vi "LVClasse_SurfaceFloat GetStatisticDatas.vi"(0 "SurfaceFloat in":refnum<class "SurfaceFloat.lvclass">, 11 "error in (no error)":errorcluster) -> (4 "SurfaceFloat out":refnum<class "SurfaceFloat.lvclass">, 6 "StatisticsData":T1, 15 "error out":errorcluster)   [LabVIEW 2020, in "SurfaceFloat.lvclass"]
doc: "Get Surface statistics.\n\n--------------------------------------------------------------------------------\n\n<B>SurfaceIn </B> : Surface object.\n<B>SurfaceOut </B> : Surface object.\n<B>rms </B> : Surface root mean square deviation.\n<B>pv </B> : Surface peak to valley.\n<B>max </B> : Surface maximum.\n<B>min </B> : Surface minimum.\n<B>ErrorIn </B> : Error\n<B>ErrorOut </B> : Error\n\n--------------------------------------------------------------------------------"
uses:
  SurfaceFloat.lvclass
  StatisticsData.ctl
  SurfaceFloat.lvclass/SurfaceFloat.ctl
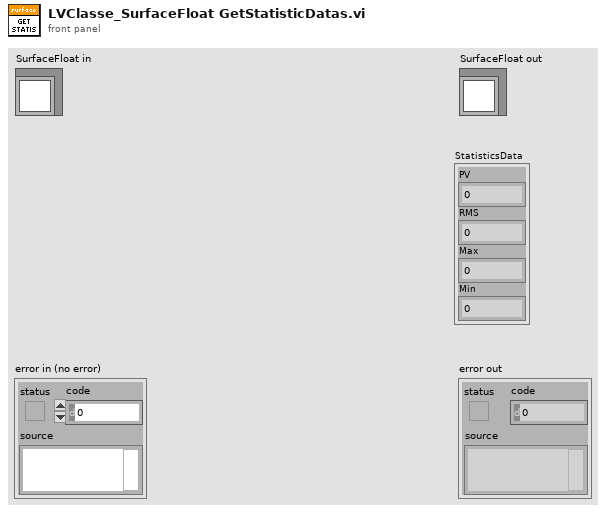
[diagram p1: front panel]
types:
  T1 = typedef "StatisticsData.ctl" = cluster{"PV":sgl, "RMS":dbl, "Max":sgl, "Min":sgl}
  T2 = typedef "ClassID.ctl" = i64
  T3 = cluster{"rms":dbl, "pv":dbl, "max":dbl, "min":dbl}
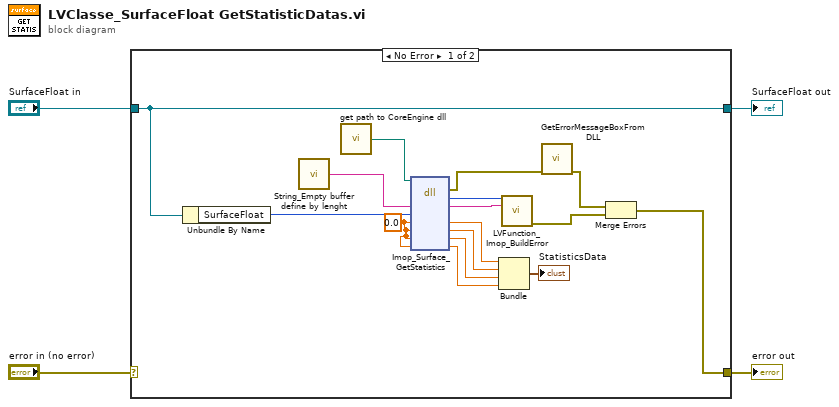
[diagram p0: block diagram]
diagram:
  n1 = case shown="No Error" "error in (no error)" {
    selector: "error in (no error)" -> [_ w22]
    tunnel: [w11 w22] -> w3
    tunnel: [w12 w21] -> w1
    tunnel: "SurfaceFloat in" -> [w12 w21]
    frame No Error {
      w10 = 0.0 ("rms")
      n2 = Unbundle By Name(w12) -> ("SurfaceFloat"=w15:T2)
      n3 = call "String_Empty buffer define by lenght.vi"() -> ("Empty buffer"=w18:string)  [unwired: 1 in]
      n4 = call "get path to CoreEngine dll.vi"() -> ("path to wavekit library"=w17:path)  [unwired: 14 in, 1 out]
      n5 = dll-call lib="D:/soft/HASO_v3/SVN_trunk/ImOpCoreEngine4_LV2011/DLLs/c_interface_vc100.dll" fn="Imop_Surface_GetStatistics"(path in=w17, "message"=w18, "surface"=w15, "rms"=w10, "pv"=w10, "max"=w10, "min"=w10) -> (error out=w16:errorcluster, "return type"=w20:i32, "message"=w19:string, "rms"=w9:dbl, "pv"=w8:dbl, "max"=w7:dbl, "min"=w6:dbl)  [unwired: 3 in, 1 out]
      n6 = Bundle("rms"=w9, "pv"=w8, "max"=w7, "min"=w6) -> (→"StatisticsData":T3)  [unwired: 1 in]
      n7 = call "LVFunction_Imop_BuildError.vi"("code"=w20, "String to Prepend to source (\"\")"=w19) -> ("error out"=w13:errorcluster)  [unwired: 13 in]
      n8 = call "GetErrorMessageBoxFromDLL.vi"("error IN"=w16) -> ("error OUT"=w14:errorcluster)  [unwired: 10 in]
      n9 = Merge Errors(w14, w13) -> (w11:errorcluster)
    }
    frame Error {
    }
  }
  "error out" <- w3
  "SurfaceFloat out" <- w1
